vi "VI.signal_control_lua.vi"(5 "LuaVIEW reference":T1) -> (15 "error out":errorcluster)   [LabVIEW 2012]
doc: "Sets the value of a front-panel control and generate a \"value changed\" event. This will cause an event structure that is monitoring the control/indicator to be signalled. Any data type that can be passed as compound data or occur as an element of compound data is supported. Useful for operating a front panel from a script, e.g. so as to perform a unit or regression test.\nParameters:\nobj:self, VI object.\nstr:label, label of control/indicator to signal.\nany:value, new value for control/indicator.\nErrors:\nNot a VI object.\nDead VI object.\nNo such control or indicator.\nData type of value does not match data type of control/indicator.\nData type of control/indicator not supported.\nCannot signal a latched boolean."
uses:
  typedefs/t_LuaVIEW Reference.ctl
  subvis/private/LuaVIEW Pull (object).vi
  subvis/private/LuaVIEW Pull (string).vi
  subvis/private/LuaVIEW Pull (flat data).vi
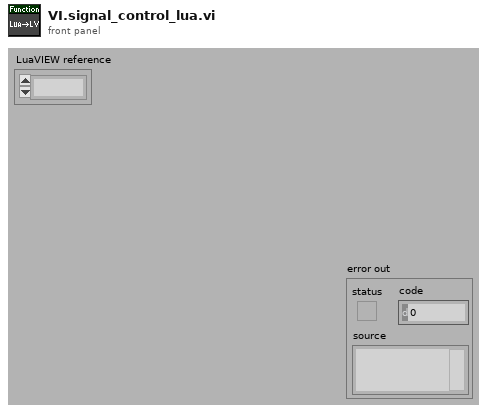
[diagram p1: front panel]
types:
  T1 = typedef "t_LuaVIEW Reference.ctl" = refnum<k1>
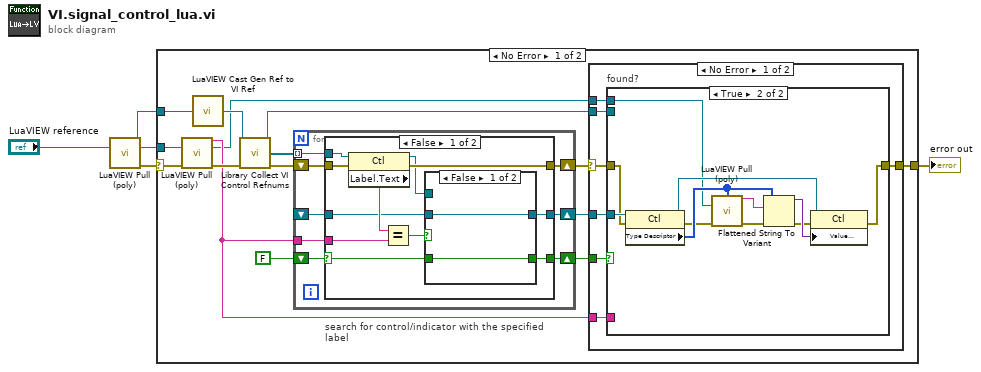
[diagram p0: block diagram]
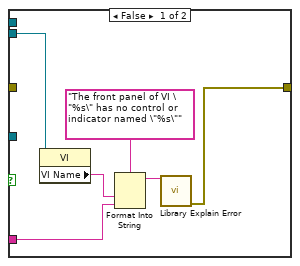
[diagram p2: hidden frame]
diagram:
  n1 = call-poly "LuaVIEW Pull (poly).vi"("LuaVIEW reference in"="LuaVIEW reference") -> ("object refnum"=w3:refnum<vi>, "LuaVIEW reference out"=w1:T1, "error out"=w2:errorcluster)  [unwired: 11 in, 1 out]
  n2 = case shown="No Error" w2 {
    selector: w2 -> [w19 w72]
    tunnel: [w6 w72] -> w4
    tunnel: w3 -> [w20 _]
    tunnel: w1 -> [w18 _]
    frame No Error {
      n3 = call-poly "LuaVIEW Pull (poly).vi"("LuaVIEW reference in"=w18, "error in (no error)"=w19) -> ("string"=w16:string, "LuaVIEW reference out"=w14:T1, "error out"=w17:errorcluster)  [unwired: 11 in]
      n4 = call "LuaVIEW Cast Gen Ref to VI Ref.vi"("refnum in"=w20) -> ("refnum out"=w15:refnum<vi>)  [unwired: 14 in]
      n5 = call "Library Collect VI Control Refnums.vi"("VI refnum in"=w15, "error in (no error)"=w17) -> ("VI refnum out"=w8:refnum<vi>, "control refnums"=w9:refnum<vi>[], "error out"=w10:errorcluster)  [unwired: 11 in]
      n6 = for "search for control/indicator with the specified label" {
        tunnel: w9 -> [w53] mode=indexing
        shift-right: [w49] -> w11
        shift-left: FALSE -> [w48]
        shift-right: [w51] -> w12
        shift-left: w10 -> [w52]
        tunnel: w16 -> [w50]
        shift-right: [w47] -> w7
        shift-left: _ -> [w46]
        n7 = case shown="False" w48 {
          selector: w48 -> [w56 w70]
          tunnel: w53 -> [w64 _]
          tunnel: w52 -> [w63 w71]
          tunnel: [w62 w71] -> w51
          tunnel: w50 -> [w60 _]
          tunnel: [w57 w70] -> w49
          tunnel: [w55 w69] -> w47
          tunnel: w46 -> [w54 w69]
          frame False {
            n8 = property class="Ctl"(reference=w64, error in=w63) -> (reference out=w58:refnum<vi>, error out=w62:errorcluster, "Label.Text"=w61:string)
            n9 = Equal?(x=w61, y=w60) -> (x = y?=w59:bool)
            n10 = case shown="False" w59 {
              selector: w59 -> [_ w68]
              tunnel: w58 -> [_ w67]
              tunnel: [w66 w68] -> w57
              tunnel: w56 -> [w66 _]
              tunnel: [w65 w67] -> w55
              tunnel: w54 -> [w65 _]
              frame False {
              }
              frame True {
              }
            }
          }
          frame True {
          }
        }
      }
      n11 = case shown="No Error" w12 {
        selector: w12 -> [w23 w45]
        tunnel: [w26 w45] -> w6
        tunnel: w11 -> [w27 _]
        tunnel: w16 -> [w25 _]
        tunnel: w8 -> [w24 _]
        tunnel: w7 -> [w22 _]
        tunnel: w14 -> [w21 _]
        frame No Error {
          n12 = case "found?" shown="True" w27 {
            tunnel: [w33 w34] -> w26
            tunnel: w25 -> [w29 _]
            tunnel: w24 -> [w32 _]
            tunnel: w23 -> [_ w35]
            tunnel: w22 -> [_ w36]
            tunnel: w21 -> [_ w37]
            frame False {
              n13 = property class="VI"(reference=w32) -> ("VI Name"=w30:string)  [unwired: 1 in, 2 out]
              n14 = Format Into String(format string="The front panel of VI \"%s\" has no control or indicator named \"%s\"", w30, w29) -> (resulting string=w31:string)  [unwired: 2 in, 1 out]
              n15 = call "Library Explain Error.vi"("explanation prefix (none)"=w31) -> ("explained error"=w33:errorcluster)  [unwired: 14 in]
            }
            frame True {
              n16 = property class="Ctl"(reference=w36, error in=w35) -> (reference out=w44:refnum<vi>, error out=w38:errorcluster, "Type Descriptor"=w39:i16[])
              n17 = call-poly "LuaVIEW Pull (poly).vi"("type descriptor"=w39, "LuaVIEW reference in"=w37, "error in (no error)"=w38) -> ("flat data"=w40:string, "error out"=w41:errorcluster)  [unwired: 10 in, 1 out]
              n18 = Flattened String To Variant(4:w41, 6:w40, 7:w39) -> (0:w42:errorcluster, 3:w43:variant)
              n19 = property class="Ctl"(reference=w44, error in=w42, "Value (Signaling)"=w43) -> (error out=w34:errorcluster)  [unwired: 1 out]
            }
          }
        }
        frame Error {
        }
      }
    }
    frame Error {
    }
  }
  "error out" <- w4
